vi "UpdateCurrentPath.vi"(8 "error in (no error)":errorcluster, 10 "Path Settings.lvclass":refnum<class "Path Settings.lvclass">, 11 "Setting Database in":refnum<class "Setting Database.lvclass">) -> (0 "error out":errorcluster, 3 "Setting Database out":refnum<class "Setting Database.lvclass">)   [LabVIEW 2020, in "Setting Database.lvclass"]
uses:
  Setting Database.lvclass
  Path Settings/Path Settings.lvclass
  C:/Users/Albro/Documents/GitHub/AFM-Lithography/lvsrc/Classes/Settings/ObjectSettings/ObjectSettings.lvclass
  C:/Users/Albro/Documents/GitHub/AFM-Lithography/lvsrc/Classes/Settings/Path Settings/Path Settings.lvclass
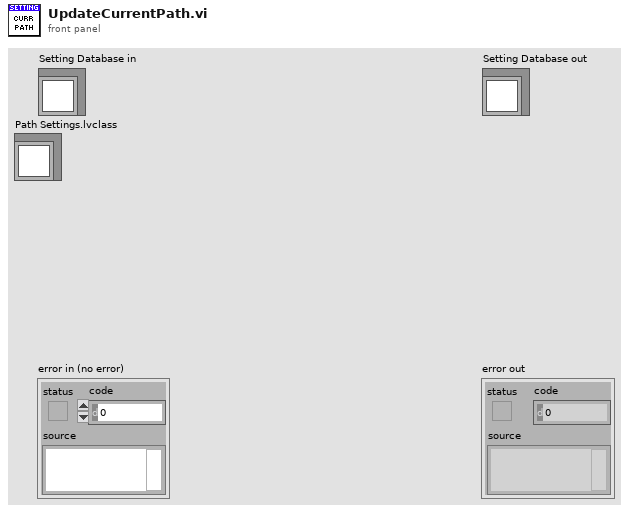
[diagram p1: front panel]
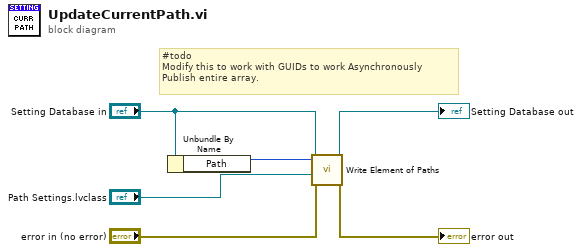
[diagram p0: block diagram]
diagram:
  # "#todo\nModify this to work with GUIDs to work Asynchronously\nPublish entire array."
  n1 = Unbundle By Name("Setting Database in") -> ("Path"=w3:i32)
  n2 = call "Write Element of Paths.vi"("error in (no error)"="error in (no error)", 9:"Path Settings.lvclass", "Path Settings.lvclass"=w3, "Setting Database in"="Setting Database in") -> ("error out"=→"error out":errorcluster, "Setting Database out"=→"Setting Database out":refnum<class "Setting Database.lvclass">)  [unwired: 6 in]
